vi "New (None).vi"(8 "error in (no error)":errorcluster, 10 "Channel Name":string) -> (0 "error out":errorcluster, 3 "Scale out":refnum<class "Scale Config.lvclass">)   [LabVIEW 2023, in "VolatusConfig.lvlib" / "Scale Config.lvclass"]
uses:
  Scale Config.lvclass
  Scale Config.lvclass/Scale Config.ctl
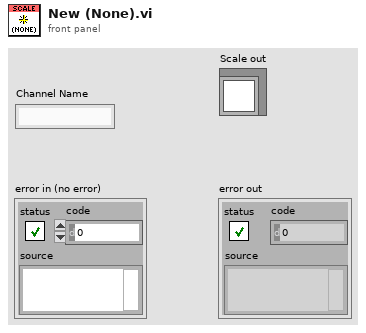
[diagram p1: front panel]
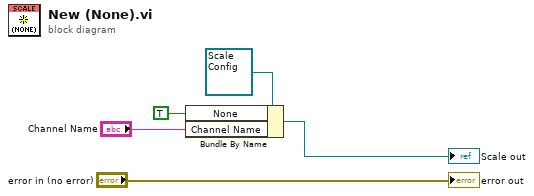
[diagram p0: block diagram]
diagram:
  n1 = Bundle By Name(cluster=refnum<class "Scale Config.lvclass"> refnum ("Scale in"), "None"=TRUE, "Channel Name"="Channel Name") -> (→"Scale out":refnum<class "Scale Config.lvclass">)
  "error out" <- "error in (no error)"
